vi "Write Display Colours.vi"(10 "Display Colours":T1, 11 "Base Display Configuration in":refnum<class "Base Display Configuration.lvclass">) -> (3 "Base Display Configuration out":refnum<class "Base Display Configuration.lvclass">)   [LabVIEW 2017, in "Assert API Components.lvlib" / "Assert Display.lvlib" / "Main Display.lvlib" / "Base Display Configuration.lvclass"]
uses:
  Base Display Configuration.lvclass
  Main Display/Display Colours.ctl
  Base Display Configuration.lvclass/Base Display Configuration.ctl
  Main Display.lvlib
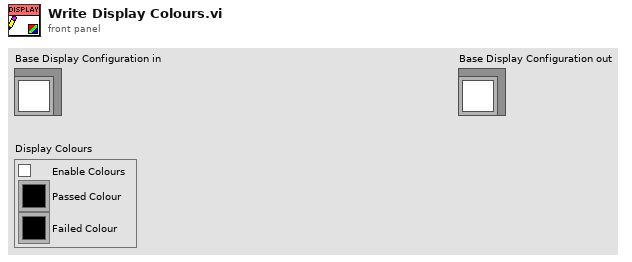
[diagram p1: front panel]
types:
  T1 = typedef "Assert API Components.lvlib/Assert Display.lvlib/Main Display.lvlib/Display Colours.ctl" = cluster{"Enable Colours":bool, "Passed Colour":u32, "Failed Colour":u32}
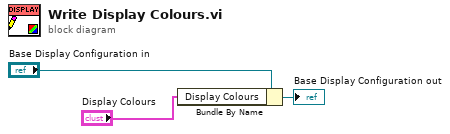
[diagram p0: block diagram]
diagram:
  n1 = Bundle By Name(cluster="Base Display Configuration in", "Display Colours"="Display Colours") -> (→"Base Display Configuration out":refnum<class "Base Display Configuration.lvclass">)
